vi "create_tweet_text.vi"(10 "controls array":refnum<vi>[](array[refnum]), 11 "time string":string) -> (3 "tweet":string="Aw yeah another whole-cell at ! #HEK")   [LabVIEW 2019]
uses:
  whole_cell_protocol/autoWC/get_data_from_control_string.vi
panel:
  out "length":i32=36
  out "number (0 to 1)":dbl=0.23779600786893917
  in  "suffix strings":string[](array[string])=[".", ". It's pretty great.", "!", " and I'm not even tired yet.", ".", ".", "!", ".", "?", "!"]
  in  "prefix strings":string[](array[string])=["Getting whole-cells in the morning, not opening the pod bay doors in the evening. ", "Look at this whole-cell I got at ", "Aw yeah another whole-cell at ", "I got a whole-cell all by myself! It's ", "Just patching, getting-whole-cells and tweeting about it. It's ", "I'm gonna give you a whole-cell you can't refuse. It's ", "I'm a neuroscience robot doing patch-clamping! Check out this cell I got at ", "Helping humanity solve the brain one whole-cell patch-clamp recording at a time. ", "What do you think about this whole-cell I got at ", "I'm a neuroscience robot recording the electrical activity of single cells! Check out this one I got at "]
  # "CREATE TWEET MESSAGE"
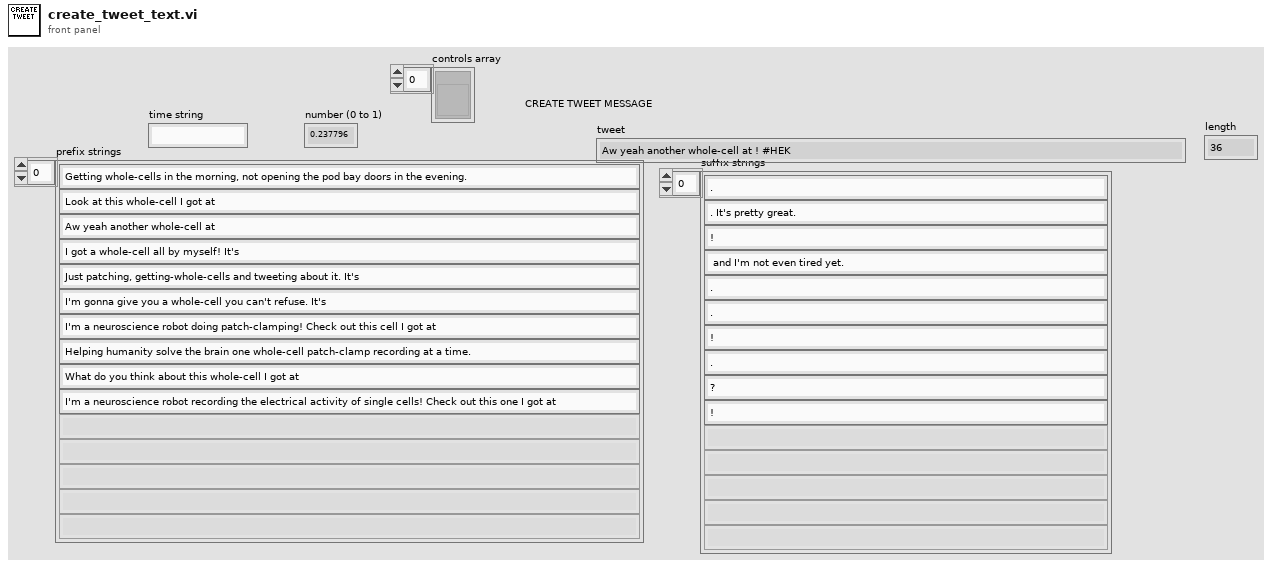
[diagram p1: front panel]
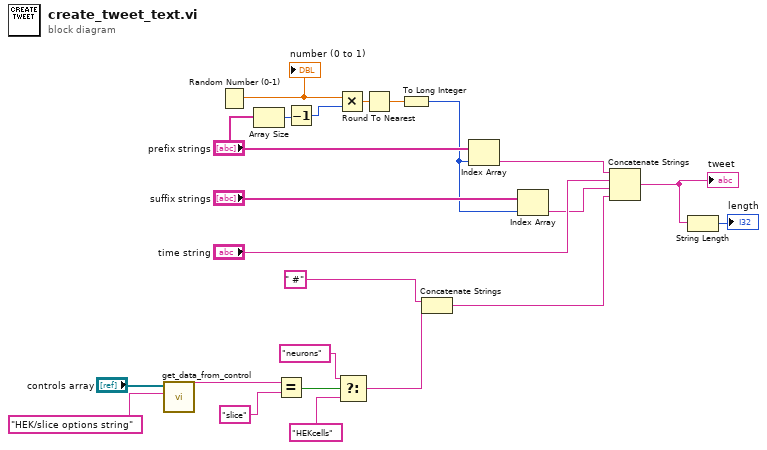
[diagram p0: block diagram]
diagram:
  n1 = call-poly "get_data_from_control.vi"("control label"="HEK/slice options string", "controls array"="controls array") -> ("string out"=w6:string)  [unwired: 8 in, 1 out]
  n2 = Random Number (0-1)() -> (number: 0 to 1=w23:dbl)
  "number (0 to 1)" <- w23
  n3 = Array Size(array="prefix strings") -> (size(s)=w14:i32)
  n4 = Equal?(x=w6, y="slice") -> (x = y?=w4:bool)
  n5 = Decrement(x=w14) -> (x-1=w13:i32)
  n6 = Multiply(x=w23, y=w13) -> (x*y=w22:dbl)
  n7 = Select(t="neurons", s=w4, f="HEKcells") -> (s? t:f=w1:string)
  n8 = Round To Nearest(number=w22) -> (nearest integer value=w21:dbl)
  n9 = To Long Integer(number=w21) -> (32bit integer=w15:i32)
  n10 = Concatenate Strings(" #", w1) -> (w7:string)
  n11 = Index Array(array="prefix strings", index=w15) -> (element=w18:string)
  n12 = Index Array(array="suffix strings", index=w15) -> (element=w16:string)
  n13 = Concatenate Strings(w18, "time string", w16, w7) -> (w12:string)
  "tweet" <- w12
  n14 = String Length(string=w12) -> (length=→"length":i32)
